vi "Handle Exceptions.vi"(8 "error in (no error)":errorcluster) -> (0 "error out":errorcluster)   [LabVIEW 2011, in "TaskbarProgressAPI.lvlib"]
doc: "This VI checks for a .Net Exception error (code 1172) and adds a note to the error source indicating that the LabVIEW Taskbar Progress Bar API may not be supported by this operating system."
uses:
  TaskbarProgressAPI.lvlib
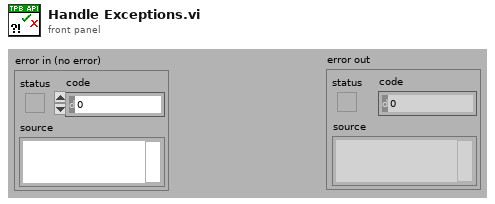
[diagram p1: front panel]
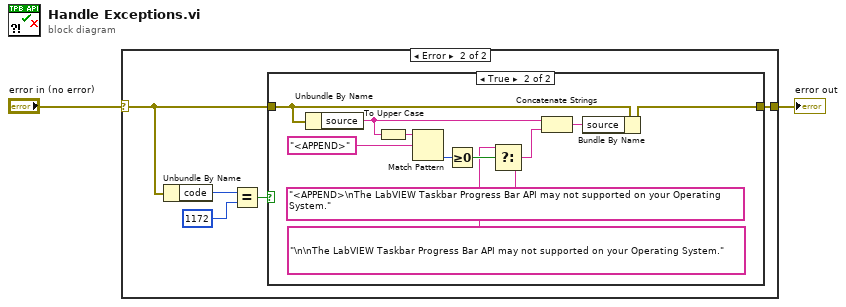
[diagram p0: block diagram]
diagram:
  n1 = case shown="Error" "error in (no error)" {
    selector: "error in (no error)" -> [w3 w5]
    tunnel: [w3 w4] -> w1
    frame No Error {
    }
    frame Error {
      n2 = Unbundle By Name(w5) -> ("code"=w8:i32)
      n3 = Equal?(x=w8, y=1172) -> (x = y?=w6:bool)
      n4 = case shown="True" w6 {
        tunnel: w5 -> [w9 w20]
        tunnel: [w9 w19] -> w4
        frame False {
        }
        frame True {
          n5 = Unbundle By Name(w20) -> ("source"=w12:string)
          n6 = To Upper Case(1:w12) -> (0:w10:string)
          n7 = Match Pattern(string=w10, regular expression="<APPEND>") -> (offset past match=w11:i32)  [unwired: 1 in, 3 out]
          n8 = Greater Or Equal To 0?(x=w11) -> (x >= 0?=w17:bool)
          n9 = Select(t="\n\nThe LabVIEW Taskbar Progress Bar API may not supported on your Operating System." ("source"), s=w17, f="<APPEND>\nThe LabVIEW Taskbar Progress Bar API may not supported on your Operating System." ("source")) -> (s? t:f=w15:string)
          n10 = Concatenate Strings(w12, w15) -> (w16:string)
          n11 = Bundle By Name(cluster=w20, "source"=w16) -> (w19:errorcluster)
        }
      }
    }
  }
  "error out" <- w1
